vi "ccc_Convert From Compatibility Conn ID.vi"(11 "old connection ID":T7) -> (3 "new connection ID":T1)   [LabVIEW 2010]
uses:
  ccc_ConnectionID.ctl
  <vilib>/NI/STM/compatibility/stm_TCP Connection Info.ctl
  <vilib>/NI/STM/compatibility/stm_MetaDataElement.ctl
  ccc_TagConfiguration.ctl
  <vilib>/NI/Current Value Table/Compatibility/_SubVIs/TypeDefs/cvt_Data Types.ctl
  ccc_TagDirection.ctl
  Connection ID.ctl
  <vilib>/NI/STM/TCP/TCP Connection Info.ctl
  <vilib>/NI/STM/SubVIs/MetaDataElement.ctl
  Tag Configuration.ctl
  <vilib>/NI/Current Value Table/Type Defs/Data Types.ctl
  Tag Direction.ctl
  <vilib>/NI/STM/NI STM.lvlib
  <vilib>/NI/Current Value Table/Current Value Table.lvlib
  NI_CCC.lvlib
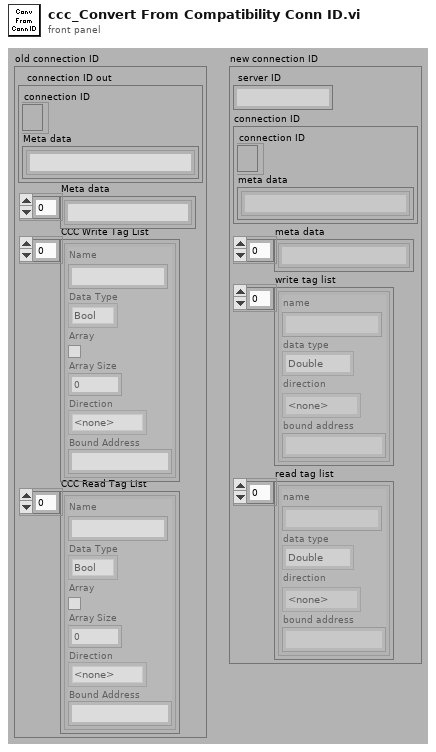
[diagram p1: front panel]
types:
  T1 = typedef "NI_CCC.lvlib/Connection ID.ctl" = cluster{"server ID":string, "connection ID":T2, "meta data":T3[], "write tag list":T4[], "read tag list":T4[]}
  T2 = typedef "NI STM.lvlib/TCP Connection Info.ctl" = cluster{"connection ID":refnum<k5>, "meta data":T3[]}
  T3 = typedef "NI STM.lvlib/MetaDataElement.ctl" = string
  T4 = typedef "NI_CCC.lvlib/Tag Configuration.ctl" = cluster{"name":string, "data type":T5, "direction":T6, "bound address":string}
  T5 = typedef "Current Value Table.lvlib/Data Types.ctl" = enum16{"Double", "Single", "I64", "I32", "I16", "I8", "U64", "U32", "U16", "U8", "String", "Boolean", "Array of U8", "Array of U16", "Array of U32", "Array of U64", "Array of I64", "Array of I32", "Array of I16", "Array of I8", "Array of Double", "Array of Single", "Array of Boolean", "Array of String"}
  T6 = typedef "NI_CCC.lvlib/Tag Direction.ctl" = enum32{"<none>", "Read", "Write"}
  T7 = typedef "ccc_ConnectionID.ctl" = cluster{"connection ID out":T8, "Meta data":T9[], "CCC Write Tag List":T10[], "CCC Read Tag List":T10[]}
  T8 = typedef "stm_TCP Connection Info.ctl" = cluster{"connection ID":refnum<k5>, "Meta data":T9[]}
  T9 = typedef "stm_MetaDataElement.ctl" = string
  T10 = typedef "ccc_TagConfiguration.ctl" = cluster{"Name":string, "Data Type":T11, "Array":bool, "Array Size":u32, "Direction":T12, "Bound Address":string}
  T11 = typedef "cvt_Data Types.ctl" = enum16{"Bool", "U8", "I32", "Double", "String", "Enum"}
  T12 = typedef "ccc_TagDirection.ctl" = enum32{"<none>", "Read", "Write"}
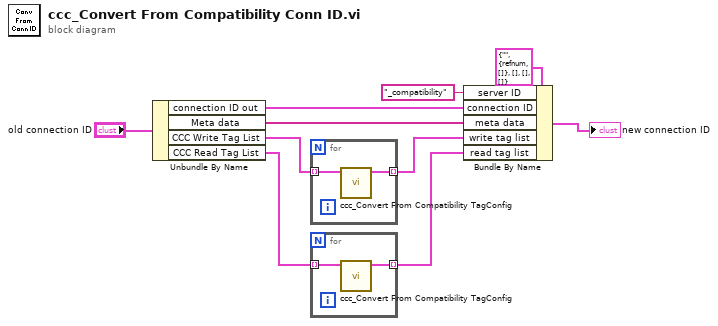
[diagram p0: block diagram]
diagram:
  n1 = Unbundle By Name("old connection ID") -> ("connection ID out"=w8:T8, "Meta data"=w7:T9[], "CCC Write Tag List"=w5:T10[], "CCC Read Tag List"=w3:T10[])
  n2 = for {
    tunnel: w5 -> [w12] mode=indexing
    tunnel: [w11] -> w4 mode=indexing
    n3 = call "ccc_Convert From Compatibility TagConfig.vi"("old tag"=w12) -> ("new tag"=w11:T4)  [unwired: 10 in]
  }
  n4 = for {
    tunnel: w3 -> [w14] mode=indexing
    tunnel: [w13] -> w2 mode=indexing
    n5 = call "ccc_Convert From Compatibility TagConfig.vi"("old tag"=w14) -> ("new tag"=w13:T4)  [unwired: 10 in]
  }
  n6 = Bundle By Name(cluster=T1 {"server ID"="", "connection ID"={"connection ID"=refnum, "meta data"=[]}, "meta data"=[], "write tag list"=[], "read tag list"=[]} ("new connection ID"), "server ID"="_compatibility", "connection ID"=w8, "meta data"=w7, "write tag list"=w4, "read tag list"=w2) -> (→"new connection ID":T1)
